vi "v2 data error mode.vi"(10 "enable_flag":bool, 11 "h":u32) -> (2 "function return":i32, 3 "h out":u32)   [LabVIEW 2019, in "apdm.lvlib"]
doc: "APDM_EXPORT int apdm_v2_data_error_mode(apdm_device_handle_t h, const bool enable_flag);"
uses:
  apdm.lvlib
  Lee Lab/CP FES Walking 2018/Code/Working/LabVIEW/apdm.dll
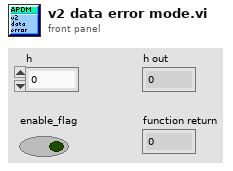
[diagram p1: front panel]
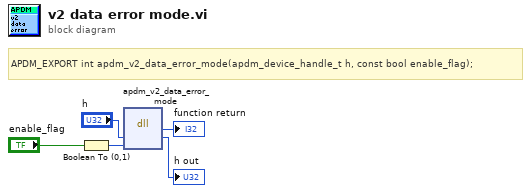
[diagram p0: block diagram]
diagram:
  # "APDM_EXPORT int apdm_v2_data_error_mode(apdm_device_handle_t h, const bool enable_flag);"
  n1 = Boolean To (0,1)(Boolean="enable_flag") -> (0, 1=w1:i16)
  n2 = dll-call lib="C:/Users/jfalesi/Dropbox/Lee Lab/CP FES Walking 2018/Code/Working/LabVIEW/apdm.*" fn="apdm_v2_data_error_mode"("h"="h", "enable_flag"=w1) -> (→"function return":i32, "h"=→"h out":u32)  [unwired: 4 in, 2 out]
